vi "Logcluster to array.vi"(0 "Log Cluster":T1, 11 "error in (no error)":errorcluster) -> (4 "Log array":string[](array[string]), 15 "error out":errorcluster)   [LabVIEW 2012]
uses:
  typedef/Log_User_Data.ctl
  typedef/User Accounts.ctl
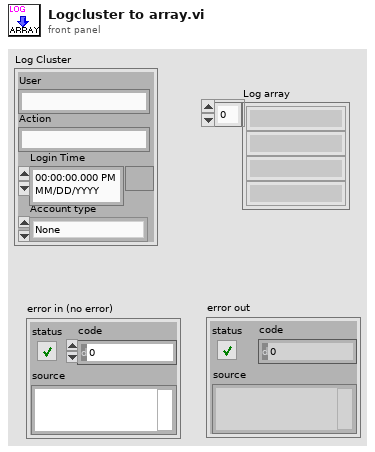
[diagram p1: front panel]
types:
  T1 = typedef "Log_User_Data.ctl" = cluster{"User":string, "Action":string, "Account type":T2, "Login Time ":timestamp}
  T2 = typedef "User Accounts.ctl" = enum16{"None", "User", "Admin"}
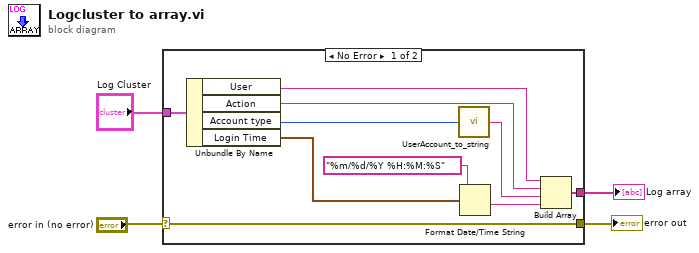
[diagram p0: block diagram]
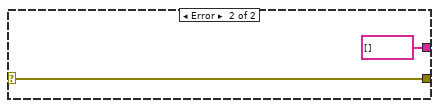
[diagram p2: hidden frame]
diagram:
  n1 = case shown="No Error" "error in (no error)" {
    selector: "error in (no error)" -> [w6 w16]
    tunnel: [w9 string[] []] -> w4
    tunnel: [w6 w16] -> w2
    tunnel: "Log Cluster" -> [w5 _]
    frame No Error {
      n2 = Unbundle By Name(w5) -> ("User"=w11:string, "Action"=w10:string, "Account type"=w12:T2, "Login Time"=w13:timestamp)
      n3 = call "UserAccount_to_string.vi"("Account"=w12) -> ("String"=w8:string)
      n4 = Format Date/Time String(time format string (%c)="%m/%d/%Y %H:%M:%S" ("format string"), seconds (now)=w13) -> (date/time string=w7:string)  [unwired: 1 in]
      n5 = Build Array(w11, w10, w8, w7) -> (w9:string[])
    }
    frame Error {
    }
  }
  "Log array" <- w4
  "error out" <- w2
